vi "shutter-control-2.vi"(7 "Wheel Speed":u8=1 min=1 max=7 step=1, 8 "error in":errorcluster, 9 "stop":bool, 10 "Laser Shutter":T1(radio), 11 "Camera Shutter":bool) -> (0 "error out":errorcluster)   [LabVIEW 2014]
uses:
  Shutter SubVis/user event shutter global.ctl
  Shutter SubVis/Global Shutter Variables - SubVI.vi
  Shutter SubVis/shutter-user-event-out-global.vi
panel:
  out "Current Wheel Position":string
  out "Status":bool
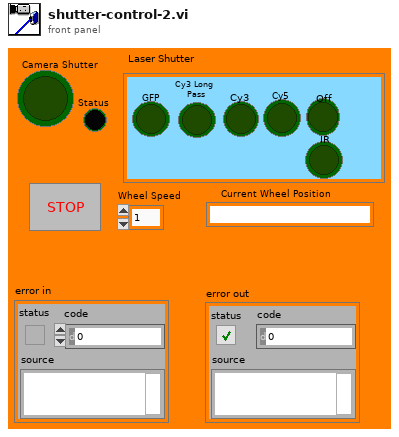
[diagram p1: front panel]
types:
  T1 = enum32{"No Selection", "GFP", "Cy3 Long \nPass", "Cy3", "Cy5", "Off", "IR"}
  T2 = typedef "user event shutter global.ctl" = cluster{"Camera Shutter":bool, "Wheel Speed":u8, "Laser Shutter":enum32{"No Selection", "GFP", "Cy3 Long \nPass", "Cy3", "Cy5", "Off", "IR"}}
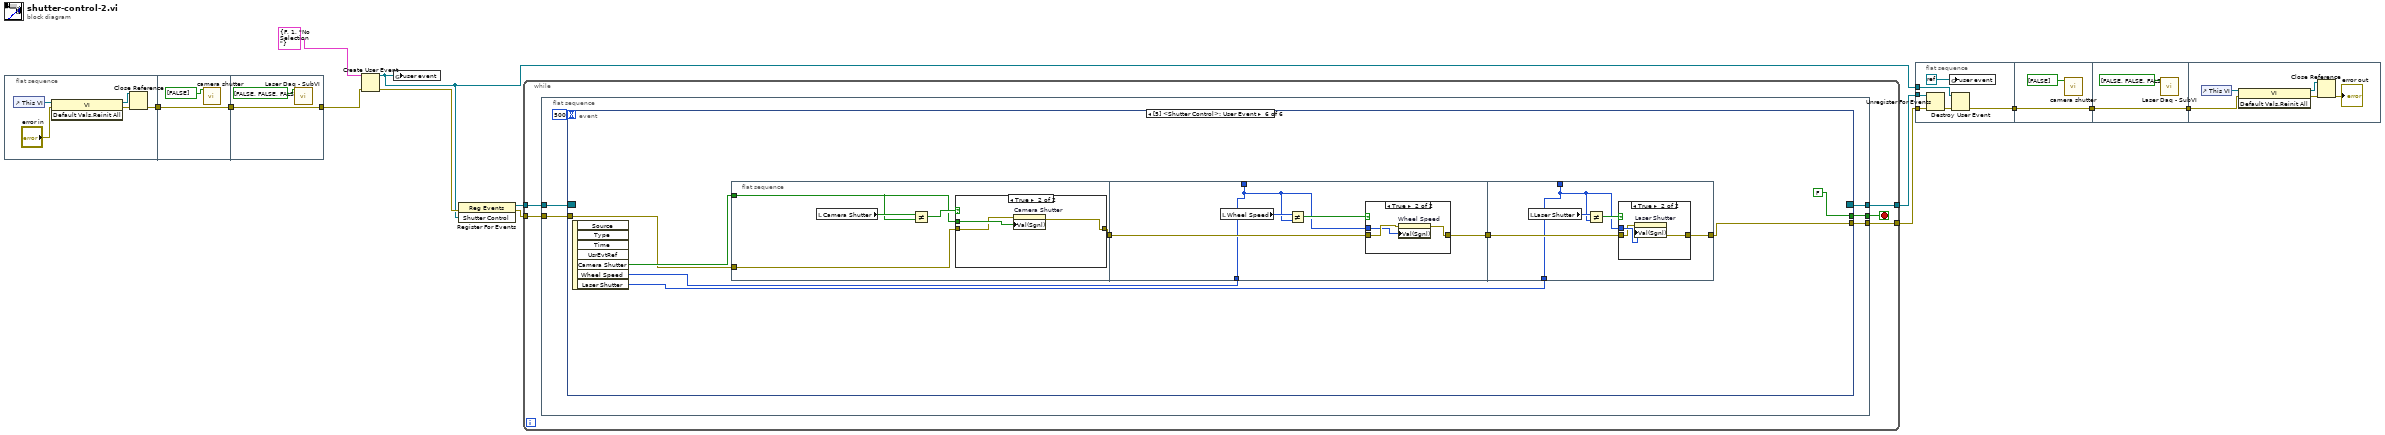
[diagram p0: block diagram]
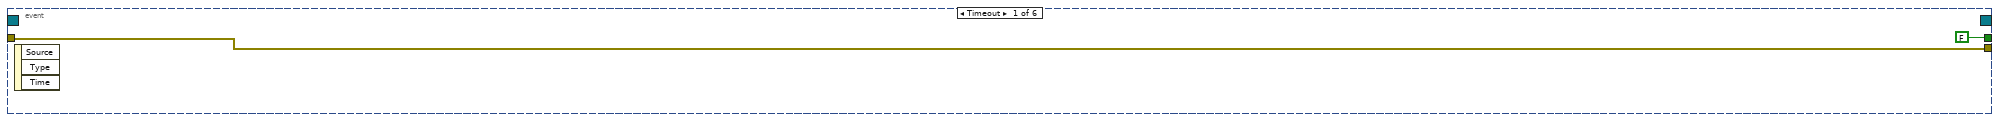
[diagram p2: hidden frame]
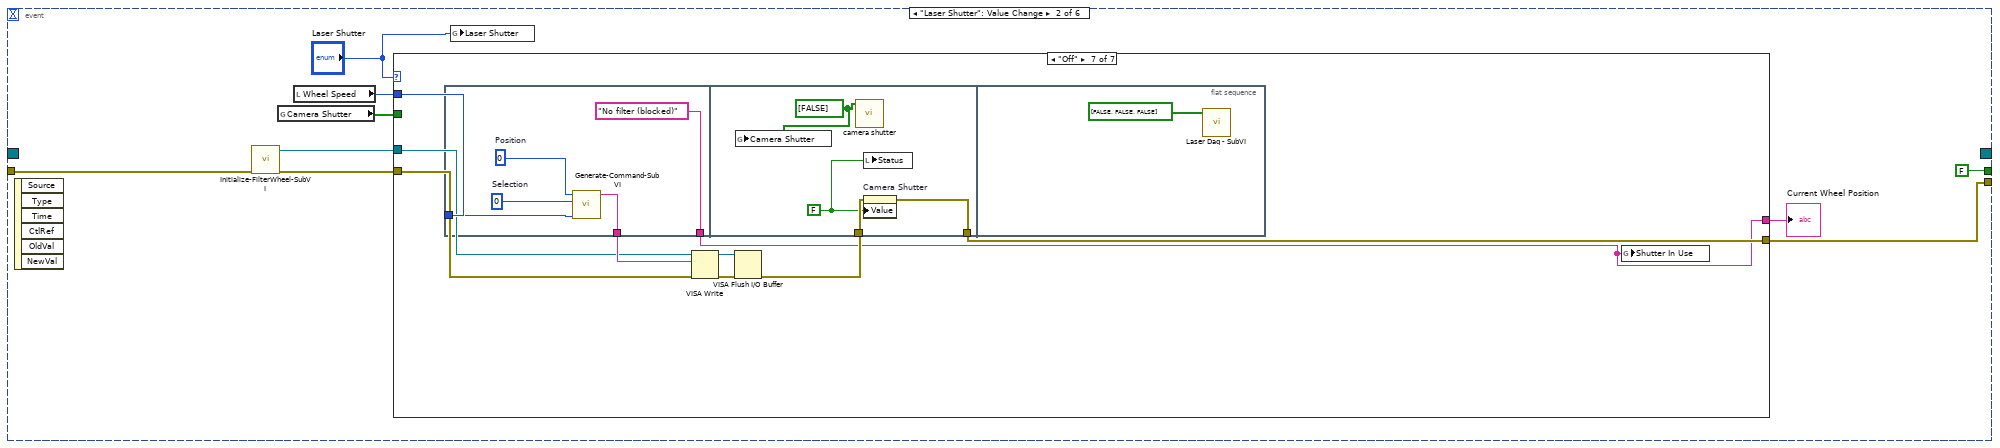
[diagram p3: hidden frame]
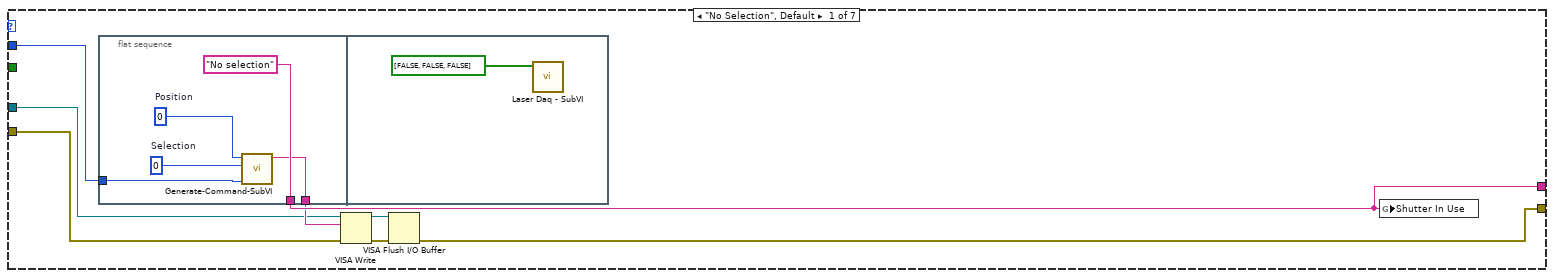
[diagram p4: hidden frame]
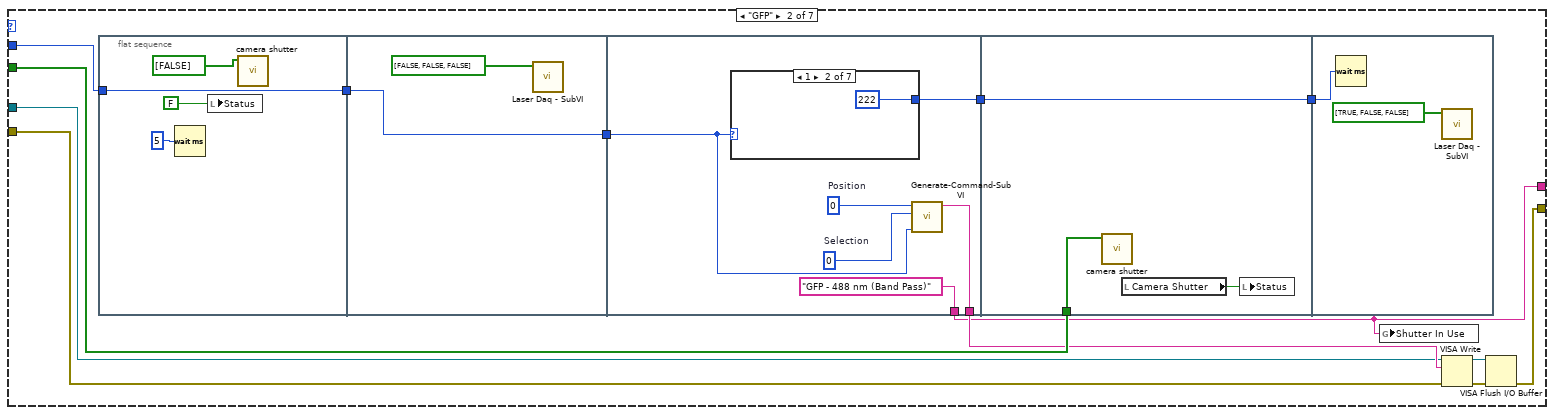
[diagram p5: hidden frame]
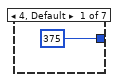
[diagram p6: hidden frame]
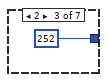
[diagram p7: hidden frame]
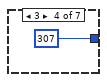
[diagram p8: hidden frame]
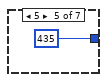
[diagram p9: hidden frame]
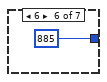
[diagram p10: hidden frame]
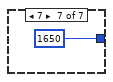
[diagram p11: hidden frame]
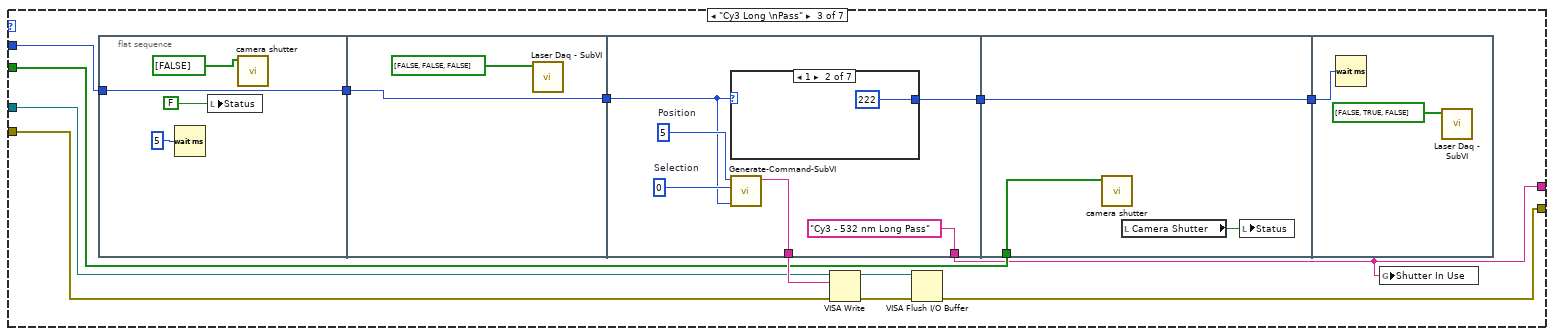
[diagram p12: hidden frame]
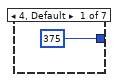
[diagram p13: hidden frame]
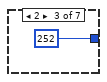
[diagram p14: hidden frame]
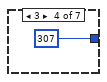
[diagram p15: hidden frame]
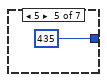
[diagram p16: hidden frame]
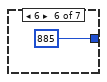
[diagram p17: hidden frame]
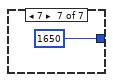
[diagram p18: hidden frame]
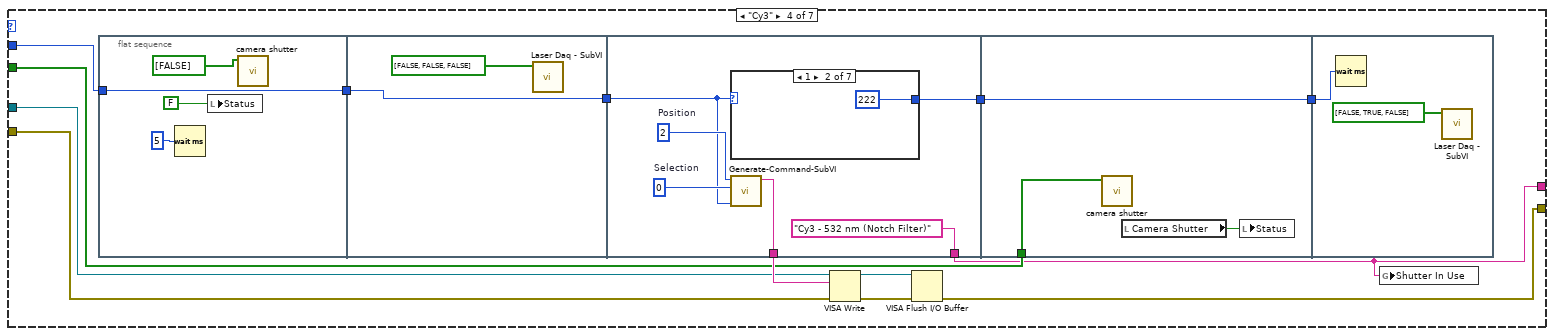
[diagram p19: hidden frame]
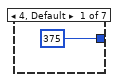
[diagram p20: hidden frame]
diagram:
  n1 = flat-sequence {
    tunnel: [w14] -> w13
    tunnel: w13 -> [w20]
    tunnel: [w20] -> w12
    tunnel: [w22] -> w7
    tunnel: w12 -> [w22]
    frame #0 {
      n2 = control-ref of="This VI"() -> (w17:refnum<vi>)
      n3 = invoke class="VI" method="Default Vals.Reinit All"(reference=w17, error in="error in") -> (reference out=w16:refnum<vi>, error out=w15:errorcluster)  [unwired: 1 in, 1 out]
      n4 = Close Reference(reference=w16, error in (no error)=w15) -> (error out=w14:errorcluster)
    }
    frame #1 {
      n5 = call "camera shutter.vi"("Array"=bool[] [FALSE]) -> ()  [unwired: 10 in, 1 out]
    }
    frame #2 {
      n6 = call "Laser Daq - SubVI.vi"("Array"=bool[] [FALSE, FALSE, FALSE]) -> ()  [unwired: 11 in]
    }
  }
  n7 = Create User Event(user event datatype=T2 {"Camera Shutter"=FALSE, "Wheel Speed"=1, "Laser Shutter"=enum."No Selection"} ("Shutter Control"), error in=w7) -> (user event=w2:refnum<user-event>, error out=w8:errorcluster)
  n8 = global write "shutter-user-event-out-global.vi" "user event"(w2) -> ()
  n9 = register-events(error in=w8, w2) -> (reference out=w5:refnum<event-registration>, error out=w6:errorcluster)  [unwired: 1 in]
  n10 = while {
    tunnel: [w27] -> w9
    tunnel: w6 -> [w24]
    tunnel: w5 -> [w25]
    tunnel: [w23] -> w3
    stop <- w26 stop-if-true
    n11 = flat-sequence {
      tunnel: w24 -> [w30]
      tunnel: w25 -> [w28]
      tunnel: [w33] -> w26
      tunnel: [w31] -> w27
      tunnel: [w29] -> w23
      frame #0 {
        n12 = event shown="[5] <Shutter Control>: User Event" {
          selector: w28 -> [_ _ _ _ _ _]
          dyn-events: [_ _ _ _ _ _] -> w29
          timeout: 500 -> [_ _ _ _ _ _]
          tunnel: [FALSE FALSE FALSE "stop" FALSE FALSE] -> w33
          tunnel: w30 -> [w34 w37 w241 w427 w430 w442]
          tunnel: [w34 w39 w239 w427 w430 w439] -> w31
          event Timeout {
            n13 = event-data() -> ()  [unwired: 1 in, 3 out]
          }
          event "Laser Shutter": Value Change {
            n14 = event-data() -> ()  [unwired: 1 in, 6 out]
            n15 = call "Initialize-FilterWheel-SubVI.vi"("error in"=w37) -> ("VISA resource name out"=w41:refnum<visa-resource-name>, "error out"=w40:errorcluster)  [unwired: 8 in]
            n16 = global read "Global Shutter Variables - SubVI.vi" "Camera Shutter"() -> (w42:bool[])
            n17 = local read "Wheel Speed"() -> (w43:u8)
            n18 = case shown="\"Off\"" "Laser Shutter" {
              tunnel: w43 -> [w51 w70 w100 w134 w174 _ w226]
              tunnel: w42 -> [_ w68 w99 w136 w172 w209 _]
              tunnel: w41 -> [w47 w64 w101 w138 w175 _ w222]
              tunnel: w40 -> [w46 w63 w98 w137 w173 w207 w221]
              tunnel: [w45 w60 w97 w135 w171 w207 w219] -> w39
              tunnel: [w52 w59 w96 w133 w170 w208 w218] -> w38
              frame "No Selection", Default {
                n19 = flat-sequence {
                  tunnel: ["No selection"] -> w52
                  tunnel: w51 -> [w54]
                  tunnel: [w53] -> w48
                  frame #0 {
                    w55 = 0  # Selection
                    w56 = 0  # Position
                    n20 = call "Generate-Command-SubVI.vi"("Wheel Speed"=w54, "Wheel Selection"=w55, "Wheel Position"=w56) -> ("type"=w53:string)  [unwired: 8 in]
                  }
                  frame #1 {
                    n21 = call "Laser Daq - SubVI.vi"("Array"=bool[] [FALSE, FALSE, FALSE]) -> ()  [unwired: 11 in]
                  }
                }
                n22 = VISA Write(VISA resource name=w47, write buffer=w48, error in (no error)=w46) -> (VISA resource name out=w49:refnum<visa-resource-name>, error out=w50:errorcluster)  [unwired: 1 out]
                n23 = VISA Flush I/O Buffer(VISA resource name=w49, error in (no error)=w50) -> (error out=w45:errorcluster)  [unwired: 1 in, 1 out]
                n24 = global write "Global Shutter Variables - SubVI.vi" "Shutter In Use"(w52) -> ()
              }
              frame "GFP" {
                n25 = flat-sequence {
                  tunnel: [w72] -> w71
                  tunnel: w70 -> [w72]
                  tunnel: w71 -> [w76]
                  tunnel: [w76] -> w69
                  tunnel: w69 -> [w81]
                  tunnel: [w80] -> w67
                  tunnel: [w79] -> w65
                  tunnel: ["GFP - 488 nm (Band Pass)"] -> w59
                  tunnel: w68 -> [w93]
                  tunnel: w67 -> [w91]
                  tunnel: [w91] -> w66
                  tunnel: w66 -> [w94]
                  frame #0 {
                    n26 = Wait (ms)(milliseconds to wait=5) -> ()  [unwired: 1 out]
                    n27 = local write "Status"(FALSE) -> ()
                    n28 = call "camera shutter.vi"("Array"=bool[] [FALSE]) -> ()  [unwired: 10 in, 1 out]
                  }
                  frame #1 {
                    n29 = call "Laser Daq - SubVI.vi"("Array"=bool[] [FALSE, FALSE, FALSE]) -> ()  [unwired: 11 in]
                  }
                  frame #2 {
                    w82 = 0  # Selection
                    w83 = 0  # Position
                    n30 = case shown="1" w81 {
                      tunnel: [375 222 252 307 435 885 1650] -> w80
                      frame 4, Default {
                      }
                      frame 1 {
                      }
                      frame 2 {
                      }
                      frame 3 {
                      }
                      frame 5 {
                      }
                      frame 6 {
                      }
                      frame 7 {
                      }
                    }
                    n31 = call "Generate-Command-SubVI.vi"("Wheel Speed"=w81, "Wheel Selection"=w82, "Wheel Position"=w83) -> ("type"=w79:string)  [unwired: 8 in]
                  }
                  frame #3 {
                    n32 = call "camera shutter.vi"("Array"=w93) -> ()  [unwired: 10 in, 1 out]
                    n33 = local read "Camera Shutter"() -> (w92:bool)
                    n34 = local write "Status"(w92) -> ()
                  }
                  frame #4 {
                    n35 = Wait (ms)(milliseconds to wait=w94) -> ()  [unwired: 1 out]
                    n36 = call "Laser Daq - SubVI.vi"("Array"=bool[] [TRUE, FALSE, FALSE]) -> ()  [unwired: 11 in]
                  }
                }
                n37 = global write "Global Shutter Variables - SubVI.vi" "Shutter In Use"(w59) -> ()
                n38 = VISA Write(VISA resource name=w64, write buffer=w65, error in (no error)=w63) -> (VISA resource name out=w62:refnum<visa-resource-name>, error out=w61:errorcluster)  [unwired: 1 out]
                n39 = VISA Flush I/O Buffer(VISA resource name=w62, error in (no error)=w61) -> (error out=w60:errorcluster)  [unwired: 1 in, 1 out]
              }
              frame "Cy3 Long \nPass" {
                n40 = flat-sequence {
                  tunnel: [w109] -> w108
                  tunnel: w100 -> [w109]
                  tunnel: w108 -> [w113]
                  tunnel: [w113] -> w107
                  tunnel: w107 -> [w118]
                  tunnel: [w117] -> w106
                  tunnel: [w116] -> w104
                  tunnel: ["Cy3 - 532 nm Long Pass"] -> w96
                  tunnel: w99 -> [w130]
                  tunnel: w106 -> [w128]
                  tunnel: [w128] -> w105
                  tunnel: w105 -> [w131]
                  frame #0 {
                    n41 = Wait (ms)(milliseconds to wait=5) -> ()  [unwired: 1 out]
                    n42 = local write "Status"(FALSE) -> ()
                    n43 = call "camera shutter.vi"("Array"=bool[] [FALSE]) -> ()  [unwired: 10 in, 1 out]
                  }
                  frame #1 {
                    n44 = call "Laser Daq - SubVI.vi"("Array"=bool[] [FALSE, FALSE, FALSE]) -> ()  [unwired: 11 in]
                  }
                  frame #2 {
                    w119 = 0  # Selection
                    w120 = 5  # Position
                    n45 = case shown="1" w118 {
                      tunnel: [375 222 252 307 435 885 1650] -> w117
                      frame 4, Default {
                      }
                      frame 1 {
                      }
                      frame 2 {
                      }
                      frame 3 {
                      }
                      frame 5 {
                      }
                      frame 6 {
                      }
                      frame 7 {
                      }
                    }
                    n46 = call "Generate-Command-SubVI.vi"("Wheel Speed"=w118, "Wheel Selection"=w119, "Wheel Position"=w120) -> ("type"=w116:string)  [unwired: 8 in]
                  }
                  frame #3 {
                    n47 = call "camera shutter.vi"("Array"=w130) -> ()  [unwired: 10 in, 1 out]
                    n48 = local read "Camera Shutter"() -> (w129:bool)
                    n49 = local write "Status"(w129) -> ()
                  }
                  frame #4 {
                    n50 = Wait (ms)(milliseconds to wait=w131) -> ()  [unwired: 1 out]
                    n51 = call "Laser Daq - SubVI.vi"("Array"=bool[] [FALSE, TRUE, FALSE]) -> ()  [unwired: 11 in]
                  }
                }
                n52 = VISA Write(VISA resource name=w101, write buffer=w104, error in (no error)=w98) -> (VISA resource name out=w103:refnum<visa-resource-name>, error out=w102:errorcluster)  [unwired: 1 out]
                n53 = VISA Flush I/O Buffer(VISA resource name=w103, error in (no error)=w102) -> (error out=w97:errorcluster)  [unwired: 1 in, 1 out]
                n54 = global write "Global Shutter Variables - SubVI.vi" "Shutter In Use"(w96) -> ()
              }
              frame "Cy3" {
                n55 = flat-sequence {
                  tunnel: [w146] -> w145
                  tunnel: w134 -> [w146]
                  tunnel: w145 -> [w150]
                  tunnel: [w150] -> w144
                  tunnel: w144 -> [w155]
                  tunnel: [w154] -> w143
                  tunnel: [w153] -> w141
                  tunnel: ["Cy3 - 532 nm (Notch Filter)"] -> w133
                  tunnel: w136 -> [w167]
                  tunnel: w143 -> [w165]
                  tunnel: [w165] -> w142
                  tunnel: w142 -> [w168]
                  frame #0 {
                    n56 = Wait (ms)(milliseconds to wait=5) -> ()  [unwired: 1 out]
                    n57 = local write "Status"(FALSE) -> ()
                    n58 = call "camera shutter.vi"("Array"=bool[] [FALSE]) -> ()  [unwired: 10 in, 1 out]
                  }
                  frame #1 {
                    n59 = call "Laser Daq - SubVI.vi"("Array"=bool[] [FALSE, FALSE, FALSE]) -> ()  [unwired: 11 in]
                  }
                  frame #2 {
                    w156 = 0  # Selection
                    w157 = 2  # Position
                    n60 = case shown="1" w155 {
                      tunnel: [375 222 252 307 435 885 1650] -> w154
                      frame 4, Default {
                      }
                      frame 1 {
                      }
                      frame 2 {
                      }
                      frame 3 {
                      }
                      frame 5 {
                      }
                      frame 6 {
                      }
                      frame 7 {
                      }
                    }
                    n61 = call "Generate-Command-SubVI.vi"("Wheel Speed"=w155, "Wheel Selection"=w156, "Wheel Position"=w157) -> ("type"=w153:string)  [unwired: 8 in]
                  }
                  frame #3 {
                    n62 = call "camera shutter.vi"("Array"=w167) -> ()  [unwired: 10 in, 1 out]
                    n63 = local read "Camera Shutter"() -> (w166:bool)
                    n64 = local write "Status"(w166) -> ()
                  }
                  frame #4 {
                    n65 = Wait (ms)(milliseconds to wait=w168) -> ()  [unwired: 1 out]
                    n66 = call "Laser Daq - SubVI.vi"("Array"=bool[] [FALSE, TRUE, FALSE]) -> ()  [unwired: 11 in]
                  }
                }
                n67 = VISA Write(VISA resource name=w138, write buffer=w141, error in (no error)=w137) -> (VISA resource name out=w140:refnum<visa-resource-name>, error out=w139:errorcluster)  [unwired: 1 out]
                n68 = VISA Flush I/O Buffer(VISA resource name=w140, error in (no error)=w139) -> (error out=w135:errorcluster)  [unwired: 1 in, 1 out]
                n69 = global write "Global Shutter Variables - SubVI.vi" "Shutter In Use"(w133) -> ()
              }
              frame "Cy5" {
                n70 = flat-sequence {
                  tunnel: [w183] -> w182
                  tunnel: w174 -> [w183]
                  tunnel: w182 -> [w188]
                  tunnel: [w188] -> w181
                  tunnel: ["Cy5 - 637 (Notch Filter)"] -> w170
                  tunnel: w181 -> [w192]
                  tunnel: [w191] -> w180
                  tunnel: [w190] -> w178
                  tunnel: w172 -> [w204]
                  tunnel: w180 -> [w202]
                  tunnel: [w202] -> w179
                  tunnel: w179 -> [w205]
                  frame #0 {
                    n71 = Wait (ms)(milliseconds to wait=5) -> ()  [unwired: 1 out]
                    n72 = local write "Status"(FALSE) -> ()
                    n73 = call "camera shutter.vi"("Array"=bool[] [FALSE]) -> ()  [unwired: 10 in, 1 out]
                  }
                  frame #1 {
                    n74 = call "Laser Daq - SubVI.vi"("Array"=bool[] [FALSE, FALSE, FALSE]) -> ()  [unwired: 11 in]
                  }
                  frame #2 {
                    w193 = 0  # Selection
                    w194 = 7  # Position
                    n75 = case shown="1" w192 {
                      tunnel: [375 222 252 307 435 885 1650] -> w191
                      frame 4, Default {
                      }
                      frame 1 {
                      }
                      frame 2 {
                      }
                      frame 3 {
                      }
                      frame 5 {
                      }
                      frame 6 {
                      }
                      frame 7 {
                      }
                    }
                    n76 = call "Generate-Command-SubVI.vi"("Wheel Speed"=w192, "Wheel Selection"=w193, "Wheel Position"=w194) -> ("type"=w190:string)  [unwired: 8 in]
                  }
                  frame #3 {
                    n77 = call "camera shutter.vi"("Array"=w204) -> ()  [unwired: 10 in, 1 out]
                    n78 = local read "Camera Shutter"() -> (w203:bool)
                    n79 = local write "Status"(w203) -> ()
                  }
                  frame #4 {
                    n80 = Wait (ms)(milliseconds to wait=w205) -> ()  [unwired: 1 out]
                    n81 = call "Laser Daq - SubVI.vi"("Array"=bool[] [FALSE, FALSE, TRUE]) -> ()  [unwired: 11 in]
                  }
                }
                n82 = global write "Global Shutter Variables - SubVI.vi" "Shutter In Use"(w170) -> ()
                n83 = VISA Write(VISA resource name=w175, write buffer=w178, error in (no error)=w173) -> (VISA resource name out=w177:refnum<visa-resource-name>, error out=w176:errorcluster)  [unwired: 1 out]
                n84 = VISA Flush I/O Buffer(VISA resource name=w177, error in (no error)=w176) -> (error out=w171:errorcluster)  [unwired: 1 in, 1 out]
              }
              frame "IR" {
                n85 = flat-sequence {
                  tunnel: [""] -> w208
                  tunnel: w209 -> [w216]
                  frame #0 {
                    n86 = local write "Status"(FALSE) -> ()
                    n87 = Wait (ms)(milliseconds to wait=5) -> ()  [unwired: 1 out]
                    n88 = call "camera shutter.vi"("Array"=bool[] [FALSE]) -> ()  [unwired: 10 in, 1 out]
                  }
                  frame #1 {
                    n89 = call "Laser Daq - SubVI.vi"("Array"=bool[] [FALSE, FALSE, FALSE]) -> ()  [unwired: 11 in]
                  }
                  frame #2 {
                  }
                  frame #3 {
                    n90 = local read "Camera Shutter"() -> (w215:bool)
                    n91 = call "camera shutter.vi"("Array"=w216) -> ()  [unwired: 10 in, 1 out]
                    n92 = local write "Status"(w215) -> ()
                  }
                  frame #4 {
                    n93 = call "Laser Daq - SubVI.vi"("Array"=bool[] [TRUE, FALSE, FALSE]) -> ()  [unwired: 11 in]
                  }
                }
              }
              frame "Off" {
                n94 = flat-sequence {
                  tunnel: w226 -> [w229]
                  tunnel: [w228] -> w223
                  tunnel: ["No filter (blocked)"] -> w218
                  tunnel: w220 -> [w235]
                  tunnel: [w234] -> w219
                  frame #0 {
                    w230 = 0  # Selection
                    w231 = 0  # Position
                    n95 = call "Generate-Command-SubVI.vi"("Wheel Speed"=w229, "Wheel Selection"=w230, "Wheel Position"=w231) -> ("type"=w228:string)  [unwired: 8 in]
                  }
                  frame #1 {
                    w232 = bool[] [FALSE]
                    w233 = FALSE
                    n96 = global write "Global Shutter Variables - SubVI.vi" "Camera Shutter"(w232) -> ()
                    n97 = call "camera shutter.vi"("Array"=w232) -> ()  [unwired: 10 in, 1 out]
                    n98 = local write "Status"(w233) -> ()
                    n99 = property on="Camera Shutter" class="Bool (strict)"(error in=w235, "Value"=w233) -> (error out=w234:errorcluster)  [unwired: 1 in, 1 out]
                  }
                  frame #2 {
                    n100 = call "Laser Daq - SubVI.vi"("Array"=bool[] [FALSE, FALSE, FALSE]) -> ()  [unwired: 11 in]
                  }
                }
                n101 = VISA Write(VISA resource name=w222, write buffer=w223, error in (no error)=w221) -> (VISA resource name out=w224:refnum<visa-resource-name>, error out=w225:errorcluster)  [unwired: 1 out]
                n102 = VISA Flush I/O Buffer(VISA resource name=w224, error in (no error)=w225) -> (error out=w220:errorcluster)  [unwired: 1 in, 1 out]
                n103 = global write "Global Shutter Variables - SubVI.vi" "Shutter In Use"(w218) -> ()
              }
            }
            "Current Wheel Position" <- w38
            n104 = global write "Global Shutter Variables - SubVI.vi" "Laser Shutter"("Laser Shutter") -> ()
          }
          event "Wheel Speed": Value Change {
            n105 = event-data() -> ()  [unwired: 1 in, 6 out]
            n106 = call "Initialize-FilterWheel-SubVI.vi"("error in"=w241) -> ("VISA resource name out"=w243:refnum<visa-resource-name>, "error out"=w242:errorcluster)  [unwired: 8 in]
            n107 = global read "Global Shutter Variables - SubVI.vi" "Camera Shutter"() -> (w240:bool[])
            n108 = local read "Laser Shutter"() -> (w244:T1)
            n109 = global write "Global Shutter Variables - SubVI.vi" "Wheel Speed"("Wheel Speed") -> ()
            n110 = case shown="\"Off\"" w244 {
              tunnel: "Wheel Speed" -> [w252 w271 w301 w335 w375 w416]
              tunnel: w240 -> [_ w269 w300 w337 w373 _]
              tunnel: w243 -> [w248 w265 w302 w339 w376 w412]
              tunnel: w242 -> [w247 w264 w299 w338 w374 w411]
              tunnel: [w246 w261 w298 w336 w372 w409] -> w239
              tunnel: [w253 w260 w297 w334 w371 w408] -> w238
              frame "No Selection", Default {
                n111 = flat-sequence {
                  tunnel: ["No selection"] -> w253
                  tunnel: w252 -> [w255]
                  tunnel: [w254] -> w249
                  frame #0 {
                    w256 = 0  # Selection
                    w257 = 0  # Position
                    n112 = call "Generate-Command-SubVI.vi"("Wheel Speed"=w255, "Wheel Selection"=w256, "Wheel Position"=w257) -> ("type"=w254:string)  [unwired: 8 in]
                  }
                  frame #1 {
                    n113 = call "Laser Daq - SubVI.vi"("Array"=bool[] [FALSE, FALSE, FALSE]) -> ()  [unwired: 11 in]
                  }
                }
                n114 = VISA Write(VISA resource name=w248, write buffer=w249, error in (no error)=w247) -> (VISA resource name out=w250:refnum<visa-resource-name>, error out=w251:errorcluster)  [unwired: 1 out]
                n115 = VISA Flush I/O Buffer(VISA resource name=w250, error in (no error)=w251) -> (error out=w246:errorcluster)  [unwired: 1 in, 1 out]
                n116 = global write "Global Shutter Variables - SubVI.vi" "Shutter In Use"(w253) -> ()
              }
              frame "GFP" {
                n117 = flat-sequence {
                  tunnel: [w273] -> w272
                  tunnel: w271 -> [w273]
                  tunnel: w272 -> [w277]
                  tunnel: [w277] -> w270
                  tunnel: w270 -> [w282]
                  tunnel: [w281] -> w268
                  tunnel: [w280] -> w266
                  tunnel: ["GFP - 488 nm (Band Pass)"] -> w260
                  tunnel: w269 -> [w294]
                  tunnel: w268 -> [w292]
                  tunnel: [w292] -> w267
                  tunnel: w267 -> [w295]
                  frame #0 {
                    n118 = Wait (ms)(milliseconds to wait=5) -> ()  [unwired: 1 out]
                    n119 = local write "Status"(FALSE) -> ()
                    n120 = call "camera shutter.vi"("Array"=bool[] [FALSE]) -> ()  [unwired: 10 in, 1 out]
                  }
                  frame #1 {
                    n121 = call "Laser Daq - SubVI.vi"("Array"=bool[] [FALSE, FALSE, FALSE]) -> ()  [unwired: 11 in]
                  }
                  frame #2 {
                    w283 = 0  # Selection
                    w284 = 0  # Position
                    n122 = case shown="1" w282 {
                      tunnel: [375 222 252 307 435 885 1650] -> w281
                      frame 4, Default {
                      }
                      frame 1 {
                      }
                      frame 2 {
                      }
                      frame 3 {
                      }
                      frame 5 {
                      }
                      frame 6 {
                      }
                      frame 7 {
                      }
                    }
                    n123 = call "Generate-Command-SubVI.vi"("Wheel Speed"=w282, "Wheel Selection"=w283, "Wheel Position"=w284) -> ("type"=w280:string)  [unwired: 8 in]
                  }
                  frame #3 {
                    n124 = call "camera shutter.vi"("Array"=w294) -> ()  [unwired: 10 in, 1 out]
                    n125 = local read "Camera Shutter"() -> (w293:bool)
                    n126 = local write "Status"(w293) -> ()
                  }
                  frame #4 {
                    n127 = Wait (ms)(milliseconds to wait=w295) -> ()  [unwired: 1 out]
                    n128 = call "Laser Daq - SubVI.vi"("Array"=bool[] [TRUE, FALSE, FALSE]) -> ()  [unwired: 11 in]
                  }
                }
                n129 = global write "Global Shutter Variables - SubVI.vi" "Shutter In Use"(w260) -> ()
                n130 = VISA Write(VISA resource name=w265, write buffer=w266, error in (no error)=w264) -> (VISA resource name out=w263:refnum<visa-resource-name>, error out=w262:errorcluster)  [unwired: 1 out]
                n131 = VISA Flush I/O Buffer(VISA resource name=w263, error in (no error)=w262) -> (error out=w261:errorcluster)  [unwired: 1 in, 1 out]
              }
              frame "Cy3 Long \nPass" {
                n132 = flat-sequence {
                  tunnel: [w310] -> w309
                  tunnel: w301 -> [w310]
                  tunnel: w309 -> [w314]
                  tunnel: [w314] -> w308
                  tunnel: w308 -> [w319]
                  tunnel: [w318] -> w307
                  tunnel: [w317] -> w305
                  tunnel: ["Cy3 - 532 nm Long Pass"] -> w297
                  tunnel: w300 -> [w331]
                  tunnel: w307 -> [w329]
                  tunnel: [w329] -> w306
                  tunnel: w306 -> [w332]
                  frame #0 {
                    n133 = Wait (ms)(milliseconds to wait=5) -> ()  [unwired: 1 out]
                    n134 = local write "Status"(FALSE) -> ()
                    n135 = call "camera shutter.vi"("Array"=bool[] [FALSE]) -> ()  [unwired: 10 in, 1 out]
                  }
                  frame #1 {
                    n136 = call "Laser Daq - SubVI.vi"("Array"=bool[] [FALSE, FALSE, FALSE]) -> ()  [unwired: 11 in]
                  }
                  frame #2 {
                    w320 = 0  # Selection
                    w321 = 5  # Position
                    n137 = case shown="1" w319 {
                      tunnel: [375 222 252 307 435 885 1650] -> w318
                      frame 4, Default {
                      }
                      frame 1 {
                      }
                      frame 2 {
                      }
                      frame 3 {
                      }
                      frame 5 {
                      }
                      frame 6 {
                      }
                      frame 7 {
                      }
                    }
                    n138 = call "Generate-Command-SubVI.vi"("Wheel Speed"=w319, "Wheel Selection"=w320, "Wheel Position"=w321) -> ("type"=w317:string)  [unwired: 8 in]
                  }
                  frame #3 {
                    n139 = call "camera shutter.vi"("Array"=w331) -> ()  [unwired: 10 in, 1 out]
                    n140 = local read "Camera Shutter"() -> (w330:bool)
                    n141 = local write "Status"(w330) -> ()
                  }
                  frame #4 {
                    n142 = Wait (ms)(milliseconds to wait=w332) -> ()  [unwired: 1 out]
                    n143 = call "Laser Daq - SubVI.vi"("Array"=bool[] [FALSE, TRUE, FALSE]) -> ()  [unwired: 11 in]
                  }
                }
                n144 = VISA Write(VISA resource name=w302, write buffer=w305, error in (no error)=w299) -> (VISA resource name out=w304:refnum<visa-resource-name>, error out=w303:errorcluster)  [unwired: 1 out]
                n145 = VISA Flush I/O Buffer(VISA resource name=w304, error in (no error)=w303) -> (error out=w298:errorcluster)  [unwired: 1 in, 1 out]
                n146 = global write "Global Shutter Variables - SubVI.vi" "Shutter In Use"(w297) -> ()
              }
              frame "Cy3" {
                n147 = flat-sequence {
                  tunnel: [w347] -> w346
                  tunnel: w335 -> [w347]
                  tunnel: w346 -> [w351]
                  tunnel: [w351] -> w345
                  tunnel: w345 -> [w356]
                  tunnel: [w355] -> w344
                  tunnel: [w354] -> w342
                  tunnel: ["Cy3 - 532 nm (Notch Filter)"] -> w334
                  tunnel: w337 -> [w368]
                  tunnel: w344 -> [w366]
                  tunnel: [w366] -> w343
                  tunnel: w343 -> [w369]
                  frame #0 {
                    n148 = Wait (ms)(milliseconds to wait=5) -> ()  [unwired: 1 out]
                    n149 = local write "Status"(FALSE) -> ()
                    n150 = call "camera shutter.vi"("Array"=bool[] [FALSE]) -> ()  [unwired: 10 in, 1 out]
                  }
                  frame #1 {
                    n151 = call "Laser Daq - SubVI.vi"("Array"=bool[] [FALSE, FALSE, FALSE]) -> ()  [unwired: 11 in]
                  }
                  frame #2 {
                    w357 = 0  # Selection
                    w358 = 2  # Position
                    n152 = case shown="1" w356 {
                      tunnel: [375 222 252 307 435 885 1650] -> w355
                      frame 4, Default {
                      }
                      frame 1 {
                      }
                      frame 2 {
                      }
                      frame 3 {
                      }
                      frame 5 {
                      }
                      frame 6 {
                      }
                      frame 7 {
                      }
                    }
                    n153 = call "Generate-Command-SubVI.vi"("Wheel Speed"=w356, "Wheel Selection"=w357, "Wheel Position"=w358) -> ("type"=w354:string)  [unwired: 8 in]
                  }
                  frame #3 {
                    n154 = call "camera shutter.vi"("Array"=w368) -> ()  [unwired: 10 in, 1 out]
                    n155 = local read "Camera Shutter"() -> (w367:bool)
                    n156 = local write "Status"(w367) -> ()
                  }
                  frame #4 {
                    n157 = Wait (ms)(milliseconds to wait=w369) -> ()  [unwired: 1 out]
                    n158 = call "Laser Daq - SubVI.vi"("Array"=bool[] [FALSE, TRUE, FALSE]) -> ()  [unwired: 11 in]
                  }
                }
                n159 = VISA Write(VISA resource name=w339, write buffer=w342, error in (no error)=w338) -> (VISA resource name out=w341:refnum<visa-resource-name>, error out=w340:errorcluster)  [unwired: 1 out]
                n160 = VISA Flush I/O Buffer(VISA resource name=w341, error in (no error)=w340) -> (error out=w336:errorcluster)  [unwired: 1 in, 1 out]
                n161 = global write "Global Shutter Variables - SubVI.vi" "Shutter In Use"(w334) -> ()
              }
              frame "Cy5" {
                n162 = flat-sequence {
                  tunnel: [w384] -> w383
                  tunnel: w375 -> [w384]
                  tunnel: w383 -> [w389]
                  tunnel: [w389] -> w382
                  tunnel: ["Cy5 - 637 (Notch Filter)"] -> w371
                  tunnel: w382 -> [w393]
                  tunnel: [w392] -> w381
                  tunnel: [w391] -> w379
                  tunnel: w373 -> [w405]
                  tunnel: w381 -> [w403]
                  tunnel: [w403] -> w380
                  tunnel: w380 -> [w406]
                  frame #0 {
                    n163 = Wait (ms)(milliseconds to wait=5) -> ()  [unwired: 1 out]
                    n164 = local write "Status"(FALSE) -> ()
                    n165 = call "camera shutter.vi"("Array"=bool[] [FALSE]) -> ()  [unwired: 10 in, 1 out]
                  }
                  frame #1 {
                    n166 = call "Laser Daq - SubVI.vi"("Array"=bool[] [FALSE, FALSE, FALSE]) -> ()  [unwired: 11 in]
                  }
                  frame #2 {
                    w394 = 0  # Selection
                    w395 = 7  # Position
                    n167 = case shown="1" w393 {
                      tunnel: [375 222 252 307 435 885 1650] -> w392
                      frame 4, Default {
                      }
                      frame 1 {
                      }
                      frame 2 {
                      }
                      frame 3 {
                      }
                      frame 5 {
                      }
                      frame 6 {
                      }
                      frame 7 {
                      }
                    }
                    n168 = call "Generate-Command-SubVI.vi"("Wheel Speed"=w393, "Wheel Selection"=w394, "Wheel Position"=w395) -> ("type"=w391:string)  [unwired: 8 in]
                  }
                  frame #3 {
                    n169 = call "camera shutter.vi"("Array"=w405) -> ()  [unwired: 10 in, 1 out]
                    n170 = local read "Camera Shutter"() -> (w404:bool)
                    n171 = local write "Status"(w404) -> ()
                  }
                  frame #4 {
                    n172 = Wait (ms)(milliseconds to wait=w406) -> ()  [unwired: 1 out]
                    n173 = call "Laser Daq - SubVI.vi"("Array"=bool[] [FALSE, FALSE, TRUE]) -> ()  [unwired: 11 in]
                  }
                }
                n174 = global write "Global Shutter Variables - SubVI.vi" "Shutter In Use"(w371) -> ()
                n175 = VISA Write(VISA resource name=w376, write buffer=w379, error in (no error)=w374) -> (VISA resource name out=w378:refnum<visa-resource-name>, error out=w377:errorcluster)  [unwired: 1 out]
                n176 = VISA Flush I/O Buffer(VISA resource name=w378, error in (no error)=w377) -> (error out=w372:errorcluster)  [unwired: 1 in, 1 out]
              }
              frame "Off" {
                n177 = flat-sequence {
                  tunnel: w416 -> [w419]
                  tunnel: [w418] -> w413
                  tunnel: ["No filter (blocked)"] -> w408
                  tunnel: w410 -> [w425]
                  tunnel: [w424] -> w409
                  frame #0 {
                    w420 = 0  # Selection
                    w421 = 0  # Position
                    n178 = call "Generate-Command-SubVI.vi"("Wheel Speed"=w419, "Wheel Selection"=w420, "Wheel Position"=w421) -> ("type"=w418:string)  [unwired: 8 in]
                  }
                  frame #1 {
                    w422 = bool[] [FALSE]
                    w423 = FALSE
                    n179 = global write "Global Shutter Variables - SubVI.vi" "Camera Shutter"(w422) -> ()
                    n180 = local write "Status"(w423) -> ()
                    n181 = property on="Camera Shutter" class="Bool (strict)"(error in=w425, "Value"=w423) -> (error out=w424:errorcluster)  [unwired: 1 in, 1 out]
                    n182 = call "camera shutter.vi"("Array"=w422) -> ()  [unwired: 10 in, 1 out]
                  }
                  frame #2 {
                    n183 = call "Laser Daq - SubVI.vi"("Array"=bool[] [FALSE, FALSE, FALSE]) -> ()  [unwired: 11 in]
                  }
                }
                n184 = VISA Write(VISA resource name=w412, write buffer=w413, error in (no error)=w411) -> (VISA resource name out=w414:refnum<visa-resource-name>, error out=w415:errorcluster)  [unwired: 1 out]
                n185 = VISA Flush I/O Buffer(VISA resource name=w414, error in (no error)=w415) -> (error out=w410:errorcluster)  [unwired: 1 in, 1 out]
                n186 = global write "Global Shutter Variables - SubVI.vi" "Shutter In Use"(w408) -> ()
              }
            }
            n187 = local write "Current Wheel Position"(w238) -> ()
          }
          event "stop": Value Change {
            n188 = event-data() -> ()  [unwired: 1 in, 6 out]
          }
          event "Camera Shutter": Value Change {
            n189 = event-data() -> ()  [unwired: 1 in, 6 out]
            n190 = global write "Global Shutter Variables - SubVI.vi" "Camera Shutter 2"("Camera Shutter") -> ()
            n191 = case shown="False" "Camera Shutter" {
              frame False {
                n192 = local write "Status"(FALSE) -> ()
                n193 = call "camera shutter.vi"("Array"=bool[] [FALSE]) -> ("Array 2"=w434:bool[])  [unwired: 10 in]
                n194 = global write "Global Shutter Variables - SubVI.vi" "Camera Shutter"(w434) -> ()
              }
              frame True {
                n195 = call "camera shutter.vi"("Array"=bool[] [TRUE]) -> ("Array 2"=w436:bool[])  [unwired: 10 in]
                n196 = global write "Global Shutter Variables - SubVI.vi" "Camera Shutter"(w436) -> ()
                "Status" <- TRUE
              }
            }
          }
          event User Event {
            n197 = event-data() -> ("Camera Shutter"=w443:bool, "Wheel Speed"=w441:u8, "Laser Shutter"=w440:T1)  [unwired: 1 in, 4 out]
            n198 = flat-sequence {
              tunnel: w443 -> [w448]
              tunnel: w442 -> [w447]
              tunnel: [w446] -> w445
              tunnel: [w455] -> _
              tunnel: w445 -> [w457]
              tunnel: [w456] -> w444
              tunnel: w441 -> [w455]
              tunnel: w444 -> [w468]
              tunnel: [w464] -> _
              tunnel: [w465] -> w439
              tunnel: w440 -> [w464]
              frame #0 {
                n199 = local read "Camera Shutter"() -> (w450:bool)
                n200 = Not Equal?(x=w450, y=w448) -> (x != y?=w449:bool)
                n201 = case shown="True" w449 {
                  tunnel: w448 -> [_ w454]
                  tunnel: w447 -> [w451 w453]
                  tunnel: [w451 w452] -> w446
                  frame False {
                  }
                  frame True {
                    n202 = property on="Camera Shutter" class="Bool (strict)"(error in=w453, "Val(Sgnl)"=w454) -> (error out=w452:errorcluster)  [unwired: 1 in, 1 out]
                  }
                }
              }
              frame #1 {
                n203 = local read "Wheel Speed"() -> (w459:u8)
                n204 = Not Equal?(x=w459, y=w455) -> (x != y?=w458:bool)
                n205 = case shown="True" w458 {
                  tunnel: w455 -> [_ w462]
                  tunnel: w457 -> [w460 w463]
                  tunnel: [w460 w461] -> w456
                  frame False {
                  }
                  frame True {
                    n206 = property on="Wheel Speed" class="DigNum (strict)"(error in=w463, "Val(Sgnl)"=w462) -> (error out=w461:errorcluster)  [unwired: 1 in, 1 out]
                  }
                }
              }
              frame #2 {
                n207 = local read "Laser Shutter"() -> (w467:T1)
                n208 = Not Equal?(x=w467, y=w464) -> (x != y?=w466:bool)
                n209 = case shown="True" w466 {
                  tunnel: w468 -> [w469 w471]
                  tunnel: w464 -> [_ w472]
                  tunnel: [w469 w470] -> w465
                  frame False {
                  }
                  frame True {
                    n210 = property on="Laser Shutter" class="RadioBtnsControl (strict)"(error in=w471, "Val(Sgnl)"=w472) -> (error out=w470:errorcluster)  [unwired: 1 in, 1 out]
                  }
                }
              }
            }
          }
        }
      }
    }
  }
  n211 = flat-sequence {
    tunnel: w9 -> [w476]
    tunnel: [w475] -> w4
    tunnel: w2 -> [w474]
    tunnel: w3 -> [w473]
    tunnel: [w479] -> w11
    tunnel: w4 -> [w479]
    tunnel: w11 -> [w481]
    tunnel: [w481] -> w10
    tunnel: w10 -> [w484]
    frame #0 {
      n212 = Unregister For Events(event registration refnum=w473, error in=w476) -> (error out=w478:errorcluster)
      n213 = global write "shutter-user-event-out-global.vi" "user event"(refnum<k0> refnum) -> ()
      n214 = Destroy User Event(user event=w474, error in=w478) -> (error out=w475:errorcluster)
    }
    frame #1 {
      n215 = call "camera shutter.vi"("Array"=bool[] [FALSE]) -> ()  [unwired: 10 in, 1 out]
    }
    frame #2 {
      n216 = call "Laser Daq - SubVI.vi"("Array"=bool[] [FALSE, FALSE, FALSE]) -> ()  [unwired: 11 in]
    }
    frame #3 {
      n217 = control-ref of="This VI"() -> (w483:refnum<vi>)
      n218 = invoke class="VI" method="Default Vals.Reinit All"(reference=w483, error in=w484) -> (reference out=w486:refnum<vi>, error out=w487:errorcluster)  [unwired: 1 in, 1 out]
      n219 = Close Reference(reference=w486, error in (no error)=w487) -> (error out=→"error out":errorcluster)
    }
  }
